vi "Read Static Child Messenger.vi"(8 "error in (no error)":errorcluster, 11 "Node Actor in":refnum<class "Node Actor.lvclass">) -> (0 "error out":errorcluster, 2 "Static System Messenger":refnum<class "Messenger.lvclass">, 3 "Node Actor out":refnum<class "Node Actor.lvclass">)   [LabVIEW 2024, in "Node Actor.lvclass"]
uses:
  Node Actor.lvclass
  C:/Users/iio/Desktop/Bussiness/Tricorn Re/Madelbrot 4.0/General Library/Ancestor Class/Actor/Root Actor/Root Actor.lvclass
  Messenger/Messenger/Messenger.lvclass
  Root Actor/Root Actor.lvclass/Root Actor.ctl
  Root Actor/Protected Data/Read Static System Messenger.vi
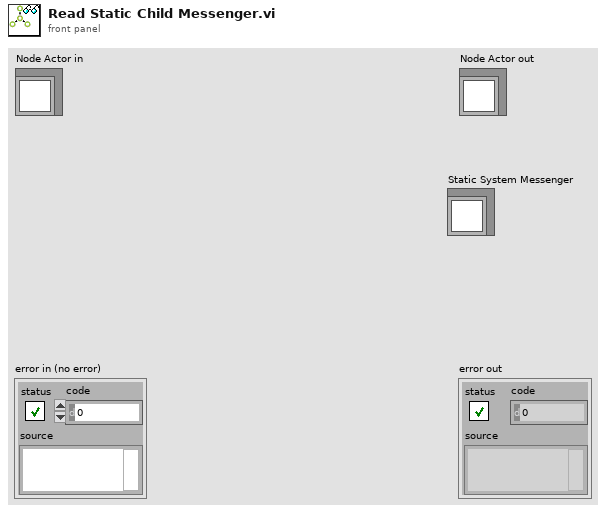
[diagram p1: front panel]
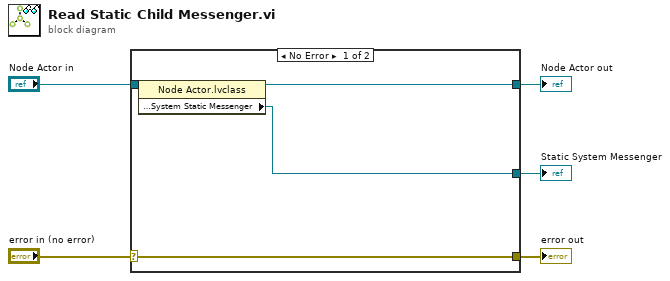
[diagram p0: block diagram]
diagram:
  n1 = case shown="No Error" "error in (no error)" {
    selector: "error in (no error)" -> [w9 w10]
    tunnel: [w9 w10] -> w4
    tunnel: [w7 w11] -> w2
    tunnel: "Node Actor in" -> [w8 w11]
    tunnel: [w6 _] -> w1
    frame No Error {
      n2 = property class="Node Actor.lvclass"(reference=w8) -> (reference out=w7:refnum<class "Node Actor.lvclass">, "Protected Data:System Static Messenger"=w6:refnum<class "Messenger.lvclass">)  [unwired: 1 in, 1 out]
    }
    frame Error {
    }
  }
  "error out" <- w4
  "Node Actor out" <- w2
  "Static System Messenger" <- w1
